vi "Max Block Count.vi"(8 "error in (no error)":errorcluster, 10 "previous block count (0)":u64, 11 "Transfer in":refnum<class "Transfer.lvclass">) -> (0 "error out":errorcluster, 2 "largest block count":u64, 3 "Transfer out":refnum<class "Transfer.lvclass">)   [LabVIEW 2017, in "DSF Core.lvlib" / "Transfer.lvclass"]
uses:
  Transfer.lvclass
  Transfer.lvclass/Transfer.ctl
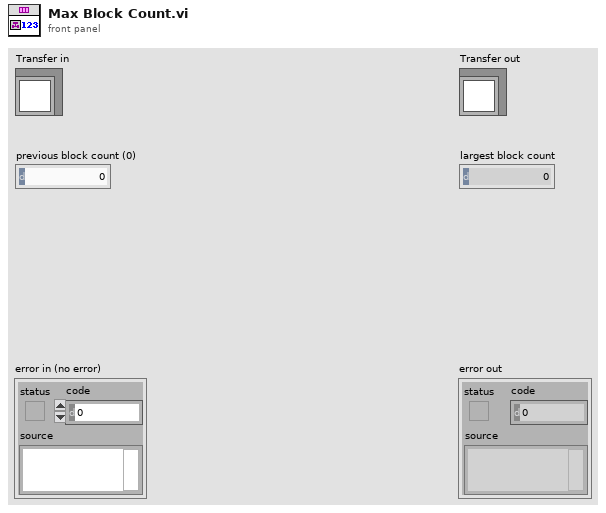
[diagram p1: front panel]
types:
  T1 = typedef "DSF Core.lvlib/DSF Engine Channel Configuration.ctl" = cluster{"src buffer offset":u64, "name":string, "data type":T2, "count":u64, "dst buffer offset":u64}
  T2 = typedef "DSF Core.lvlib/DSF Data Type.ctl" = enum8{"Bool", "SGL", "DBL", "I8", "I16", "I32", "I64", "U8", "U16", "U32", "U64"}
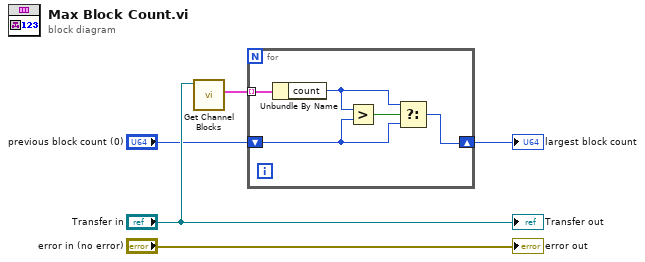
[diagram p0: block diagram]
diagram:
  n1 = call "Get Channel Blocks.vi"("Transfer in"="Transfer in") -> ("channel blocks"=w3:T1[])  [unwired: 9 in, 1 out]
  n2 = for {
    tunnel: w3 -> [w10] mode=indexing
    shift-right: [w6] -> w1
    shift-left: "previous block count (0)" -> [w7]
    n3 = Unbundle By Name(w10) -> ("count"=w8:u64)
    n4 = Greater?(x=w8, y=w7) -> (0:w9:bool)
    n5 = Select(t=w8, s=w9, f=w7) -> (s? t:f=w6:u64)
  }
  "largest block count" <- w1
  "error out" <- "error in (no error)"
  "Transfer out" <- "Transfer in"
